vi "libssh2_init (Custom).vi"(8 "error in (no error)":errorcluster, 11 "path (use built-in)":path) -> (0 "error out":errorcluster)   [LabVIEW 2013, in "libssh2.lvlib"]
doc: "Initializes libssh2 using the library specified by <B>path</B>."
uses:
  libssh2.lvlib
  Global Settings.vi
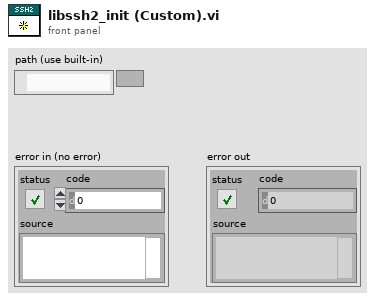
[diagram p1: front panel]
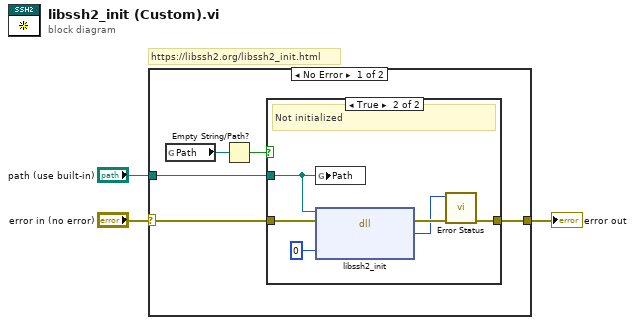
[diagram p0: block diagram]
diagram:
  # "https://libssh2.org/libssh2_init.html"
  n1 = case shown="No Error" "error in (no error)" {
    selector: "error in (no error)" -> [w7 w16]
    tunnel: [w8 w16] -> w3
    tunnel: "path (use built-in)" -> [w6 _]
    frame No Error {
      n2 = global read "Global Settings.vi" "Path"() -> (w4:path)
      n3 = Empty String/Path?(string/path=w4) -> (empty?=w5:bool)
      n4 = case shown="True" w5 {
        tunnel: [w9 w11] -> w8
        tunnel: w7 -> [w9 w13]
        tunnel: w6 -> [_ w12]
        frame False {
          # "Already initialized"
        }
        frame True {
          # "Not initialized"
          n5 = global write "Global Settings.vi" "Path"(w12) -> ()
          n6 = dll-call lib="C:/Users/pasca/source/repos/libssh2-labview/libssh2/libssh2**.*" fn="libssh2_init"(path in=w12, error in=w13, "flags"=0) -> (error out=w14:errorcluster, "return value"=w10:i32)  [unwired: 2 in, 1 out]
          n7 = call "Error Status.vi"("error in (no error)"=w14, "return value"=w10) -> ("error out"=w11:errorcluster)  [unwired: 9 in]
        }
      }
    }
    frame Error {
    }
  }
  "error out" <- w3
